vi "magnetic-field.vi"(3 "dist to goal nullify":dbl=200.0, 5 "max angle (greater)":dbl=1.1 format="%#_13g", 6 "max force":dbl=3.0 format="%#_13g", 7 "enemy influence radius":dbl=700.0 format="%#_13g", 8 "goal pos":dbl[](array[numeric])=[0.0, 0.0] format="%#_13g", 9 "enemy pos":dbl[](array[numeric])=[0.0, 1e-10] format="%#_13g", 11 "ally pos":dbl[](array[numeric])=[0.0, 0.0] format="%#_13g") -> (2 "magnetic force":dbl[](array[numeric]))   [LabVIEW 2017]
uses:
  <vilib>/Analysis/_algsub.llb/Vector Norm Type.ctl
  <vilib>/Analysis/baseanly.llb/Unit Vector (DBL).vi
  <vilib>/Analysis/NI_AALBase.lvlib
  <vilib>/Analysis/NI_AALPro.lvlib
panel:
  in  "too close":dbl=90.0 format="%#_13g"
  in  "y wrap around switch eps":dbl=20.0 format="%#_13g"
  out "magnitude":dbl
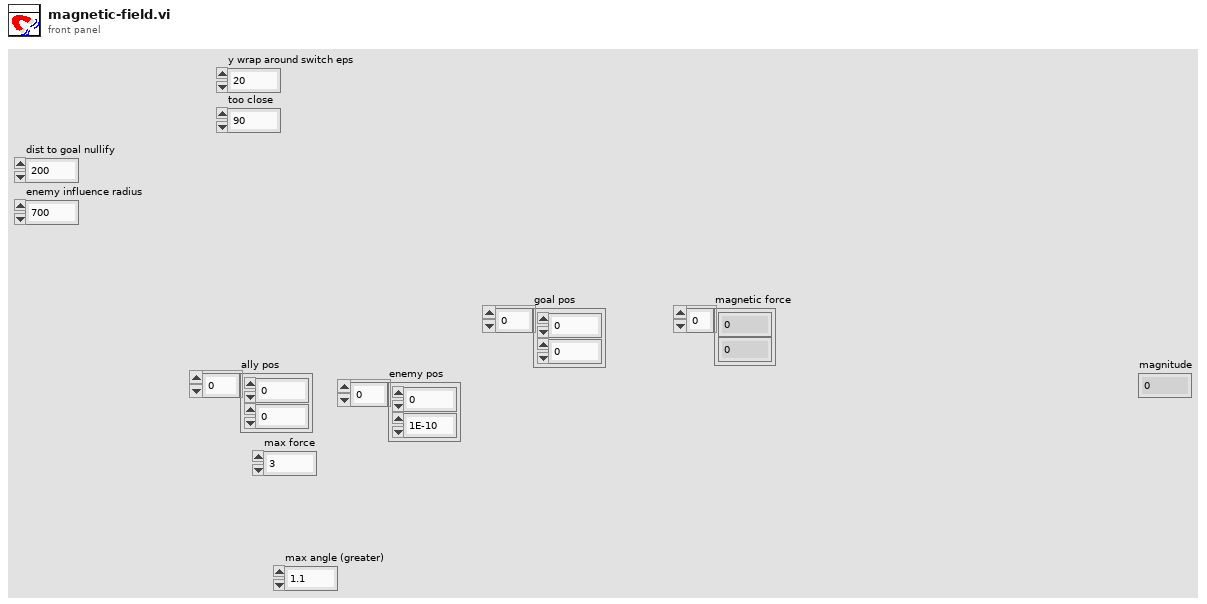
[diagram p1: front panel]
types:
  T1 = typedef "NI_AALPro.lvlib/Vector Norm Type.ctl" = u16
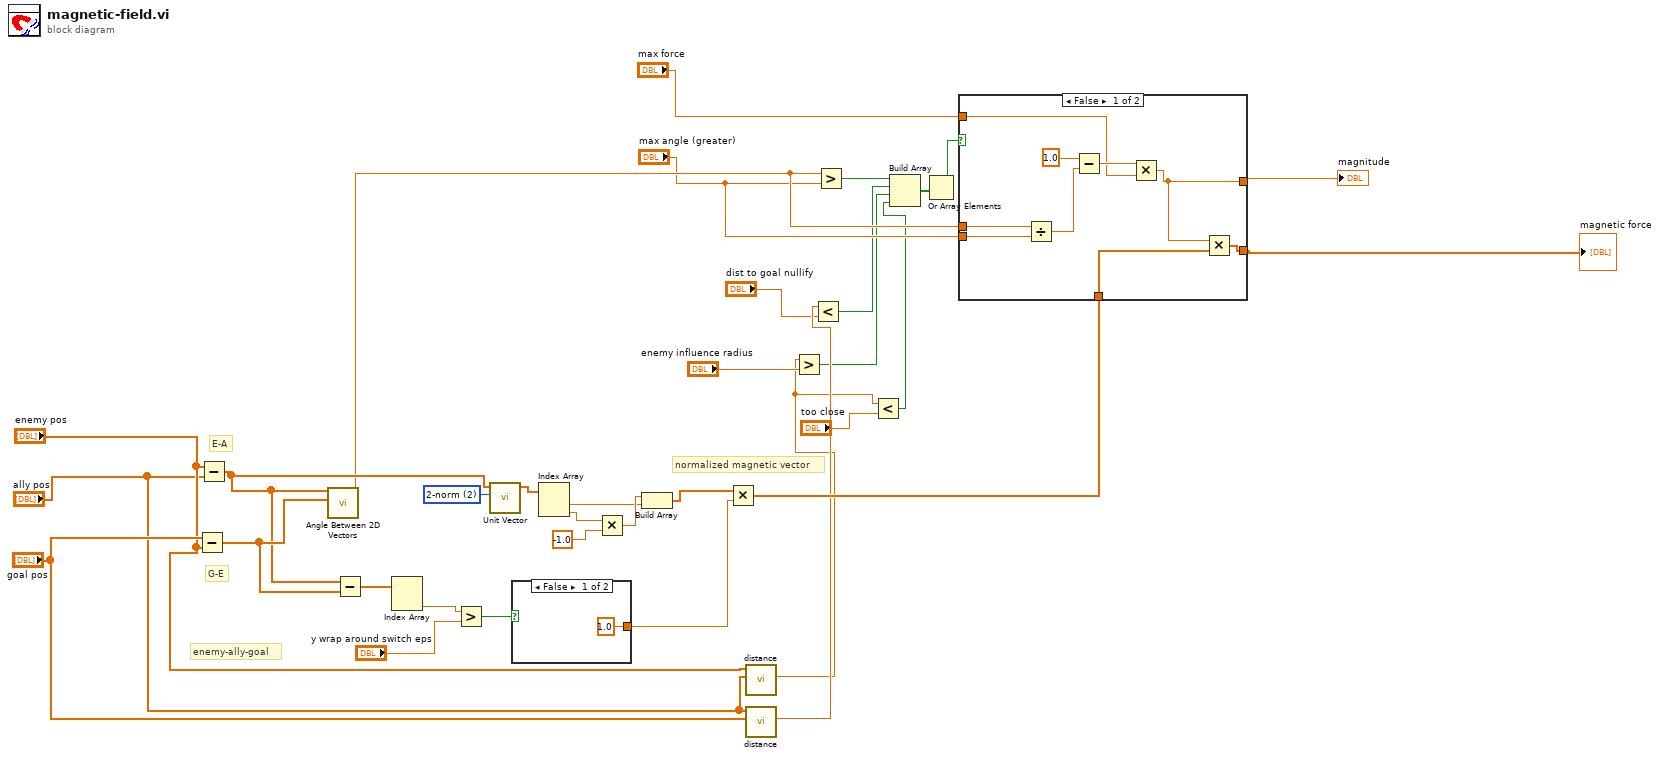
[diagram p0: block diagram]
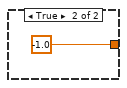
[diagram p2: hidden frame]
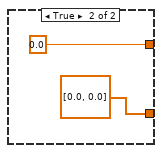
[diagram p3: hidden frame]
diagram:
  w30 = T1 2 items=["1-norm"=1, "2-norm"=2, "Inf-norm"=3, "-Inf-norm"=4, "User Defined"=5] ("norm type")
  # "normalized magnetic vector"
  # "enemy-ally-goal"
  # "E-A"
  # "G-E"
  n1 = Subtract(x="goal pos", y="enemy pos") -> (x-y=w33:dbl[])
  n2 = Subtract(x="enemy pos", y="ally pos") -> (x-y=w31:dbl[])
  n3 = call "Angle Between 2D Vectors.vi"("Array"=w33, "Array 2"=w31) -> ("Numeric"=w23:dbl)  [unwired: 9 in]
  n4 = Subtract(x=w31, y=w33) -> (x-y=w32:dbl[])
  n5 = Index Array(array=w32) -> (element #2=w20:dbl)  [unwired: 2 in, 1 out]
  n6 = Greater?(x=w20, y="y wrap around switch eps") -> (0:w18:bool)
  n7 = call-poly <vilib>:"Unit Vector.vi"("norm type"=w30, "Input Vector"=w31) -> ("Unit Vector"=w29:dbl[])  [unwired: 7 in, 2 out]
  n8 = case shown="False" w18 {
    tunnel: [1.0 ("y") -1.0 ("y")] -> w17
    frame False {
    }
    frame True {
    }
  }
  n9 = Index Array(array=w29) -> (element #1=w25:dbl, element #2=w28:dbl)  [unwired: 2 in]
  n10 = Multiply(x=w28, y=-1.0) -> (x*y=w26:dbl)
  n11 = Build Array(w26, w25) -> (w24:dbl[])
  n12 = Multiply(x=w24, y=w17) -> (x*y=w16:dbl[])
  n13 = call "distance.vi"("target pos"="ally pos", "obj pos"="enemy pos") -> ("sqrt(x)"=w3:dbl)  [unwired: 9 in]
  n14 = call "distance.vi"("target pos"="goal pos", "obj pos"="ally pos") -> ("sqrt(x)"=w13:dbl)  [unwired: 9 in]
  n15 = Greater?(x=w3, y="enemy influence radius") -> (0:w6:bool)
  n16 = Less?(x=w13, y="dist to goal nullify") -> (x < y?=w7:bool)
  n17 = Greater?(x=w23, y="max angle (greater)") -> (0:w8:bool)
  n18 = Less?(x=w3, y="too close") -> (x < y?=w1:bool)
  n19 = Build Array(w8, w7, w6, w1) -> (w5:bool[])
  n20 = Or Array Elements(Boolean array=w5) -> (logical OR=w4:bool)
  n21 = case shown="False" w4 {
    tunnel: [w38 0.0] -> w34
    tunnel: w23 -> [w45 _]
    tunnel: "max angle (greater)" -> [w43 _]
    tunnel: "max force" -> [w40 _]
    tunnel: w16 -> [w39 _]
    tunnel: [w37 dbl[] [0.0, 0.0]] -> w15
    frame False {
      n22 = Divide(x=w45, y=w43) -> (x/y=w42:dbl)
      n23 = Subtract(x=1.0, y=w42) -> (x-y=w41:dbl)
      n24 = Multiply(x=w41, y=w40) -> (x*y=w38:dbl)
      n25 = Multiply(x=w38, y=w39) -> (x*y=w37:dbl[])
    }
    frame True {
    }
  }
  "magnitude" <- w34
  "magnetic force" <- w15
